vi "Build Bulk Create Parameters.vi"(4 "TypeMap in":refnum<class "TypeMap.lvclass">, 8 "error in (no error)":errorcluster, 10 "object":variant[](array[variant]), 11 "SqlMapper in":refnum<class "SqlMapper.lvclass">) -> (0 "error out":errorcluster, 1 "DynamicParameters out":refnum<class "DynamicParameters.lvclass">[](array[class]), 3 "SqlMapper out":refnum<class "SqlMapper.lvclass">)   [LabVIEW 2020, in "ORM.lvlib" / "TypeMap.lvclass"]
uses:
  TypeMap.lvclass
  DynamicParameters/DynamicParameters.lvclass
  SqlMapper/SqlMapper.lvclass
  TypeMap.lvclass/TypeMap.ctl
  Read Autokey.vi
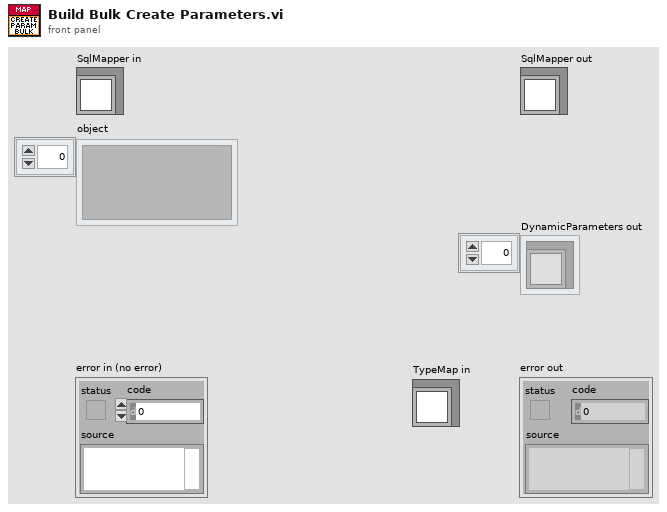
[diagram p1: front panel]
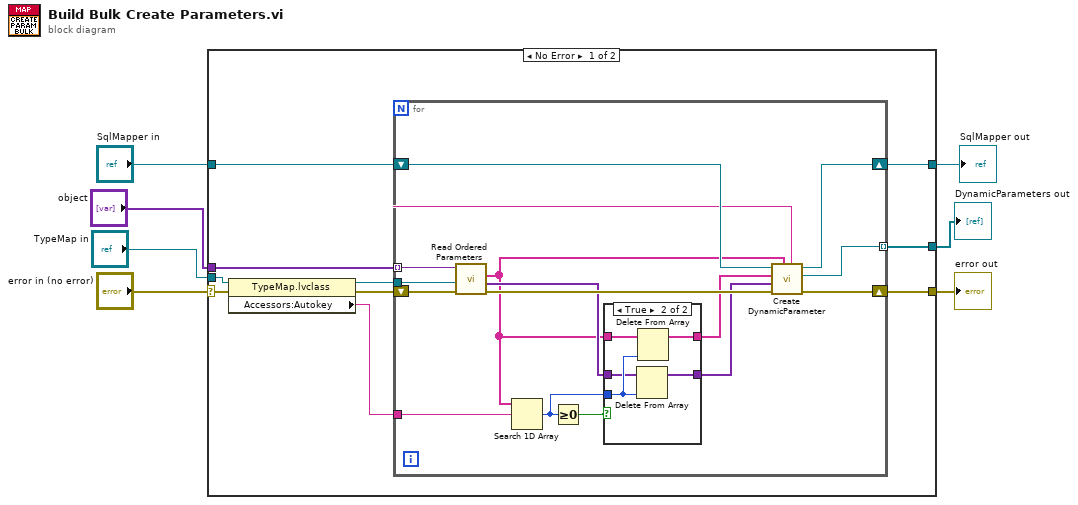
[diagram p0: block diagram]
diagram:
  n1 = case shown="No Error" "error in (no error)" {
    selector: "error in (no error)" -> [w16 w41]
    tunnel: [w12 w41] -> w6
    tunnel: "TypeMap in" -> [w17 _]
    tunnel: "object" -> [w8 _]
    tunnel: [w13 _] -> w3
    tunnel: [w14 w40] -> w2
    tunnel: "SqlMapper in" -> [w15 w40]
    frame No Error {
      n2 = property class="TypeMap.lvclass"(reference=w17, error in=w16) -> (reference out=w9:refnum<class "TypeMap.lvclass">, error out=w10:errorcluster, "Accessors:Autokey"=w11:string)
      n3 = for {
        tunnel: [w29] -> w13 mode=indexing
        tunnel: w11 -> [w23]
        tunnel: w9 -> [w21]
        tunnel: w8 -> [w20] mode=indexing
        shift-right: [w30] -> w14
        shift-left: w15 -> [w31]
        shift-right: [w24] -> w12
        shift-left: w10 -> [w22]
        n4 = call "Read Ordered Parameters.vi"("error in (no error)"=w22, "TypeMap in"=w21, "Object In"=w20) -> ("error out"=w32:errorcluster, "Values"=w19:variant[], "Fields"=w18:string[])  [unwired: 5 in, 1 out]
        n5 = Search 1D Array(1D array=w18, element=w23) -> (index of element=w27:i32)  [unwired: 1 in]
        n6 = Greater Or Equal To 0?(x=w27) -> (x >= 0?=w28:bool)
        n7 = case shown="True" w28 {
          tunnel: w27 -> [_ w39]
          tunnel: w18 -> [w34 w38]
          tunnel: w19 -> [w33 w37]
          tunnel: [w34 w36] -> w26
          tunnel: [w33 w35] -> w25
          frame False {
          }
          frame True {
            n8 = Delete From Array(array=w37, index=w39) -> (array with subset deleted=w35:variant[])  [unwired: 1 in, 1 out]
            n9 = Delete From Array(array=w38, index=w39) -> (array with subset deleted=w36:string[])  [unwired: 1 in, 1 out]
          }
        }
        n10 = call "Create DynamicParameter.vi"("AutoKey"=w23, "RequestedFields"=w18, "error in (no error)"=w32, "ParameterValues"=w25, "ParameterNames"=w26, "SqlMapper in"=w31) -> ("error out"=w24:errorcluster, "Parameters"=w29:refnum<class "DynamicParameters.lvclass">, "SqlMapper out"=w30:refnum<class "SqlMapper.lvclass">)  [unwired: 1 in, 2 out]
      }
    }
    frame Error {
    }
  }
  "error out" <- w6
  "DynamicParameters out" <- w3
  "SqlMapper out" <- w2
